vi "SNMP Open Port.vi"(8 "error in (no error)":errorcluster, 11 "port":u16) -> (0 "error out":errorcluster, 3 "connection ID":refnum<k16>)   [LabVIEW 2017]
doc: "This VI is used to open a SNMP session."
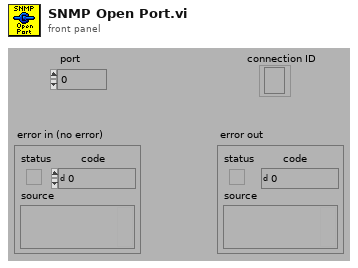
[diagram p1: front panel]
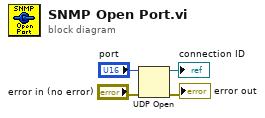
[diagram p0: block diagram]
diagram:
  n1 = UDP Open(8:"error in (no error)", 11:"port") -> (port=→"connection ID":refnum<k16>, 0:→"error out":errorcluster)  [unwired: 4 out]
